vi "LastName.vi"(2 "Custom Folder":string, 3 "Extention":string="dat", 4 "User Data Folder":path) -> (0 "created path":path, 1 "String":string)   [LabVIEW 2017]
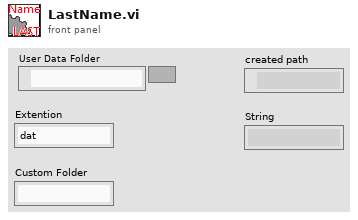
[diagram p1: front panel]
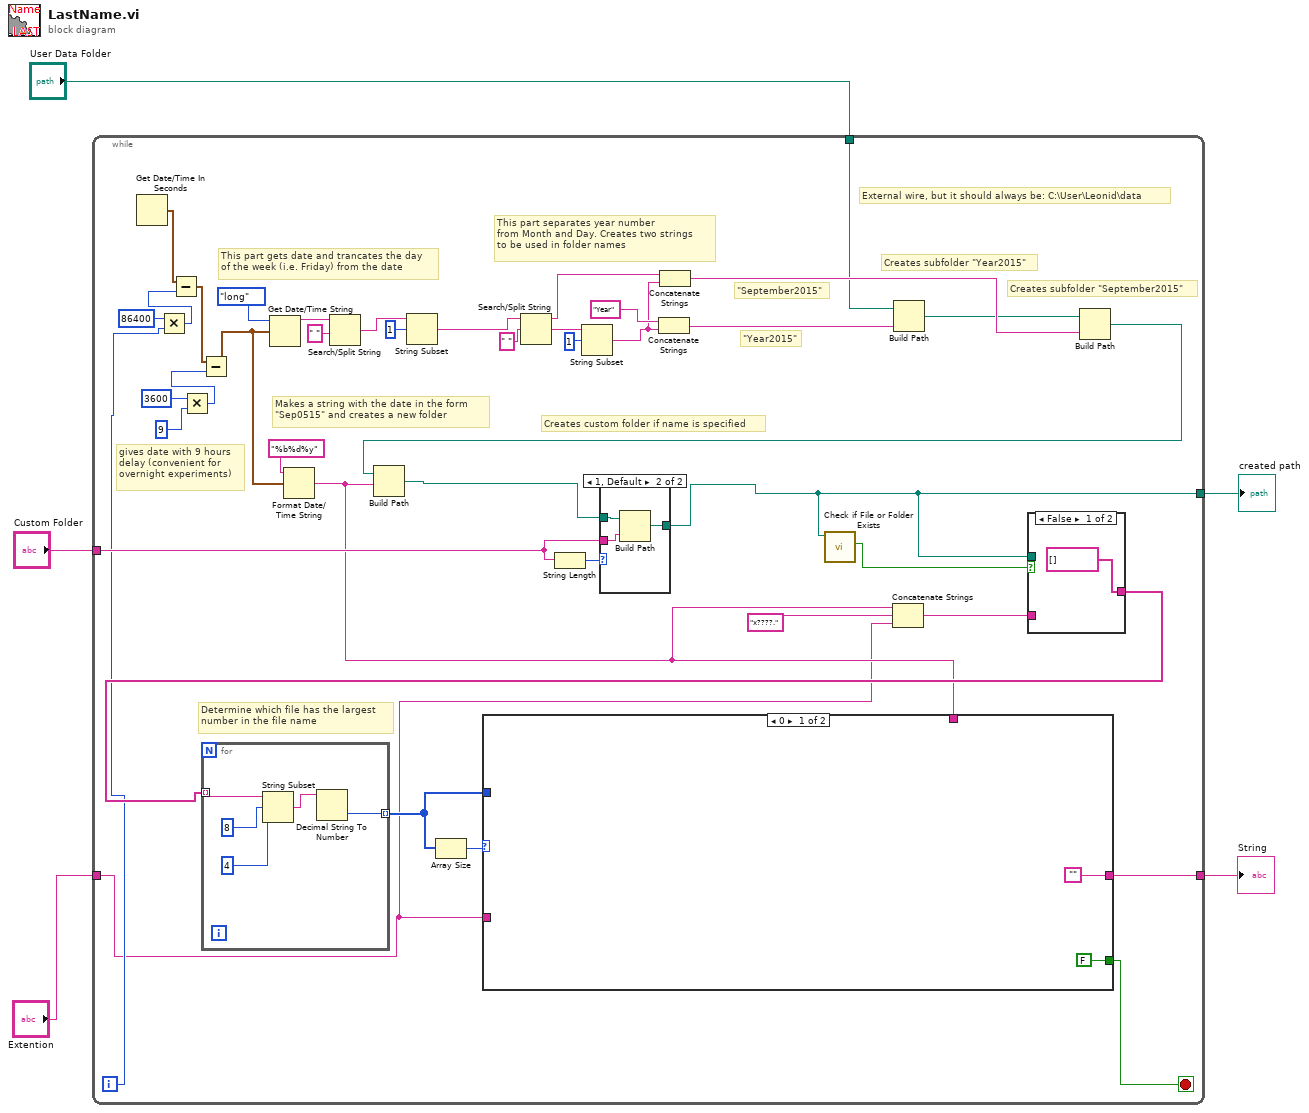
[diagram p0: block diagram]
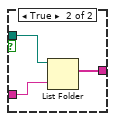
[diagram p2: hidden frame]
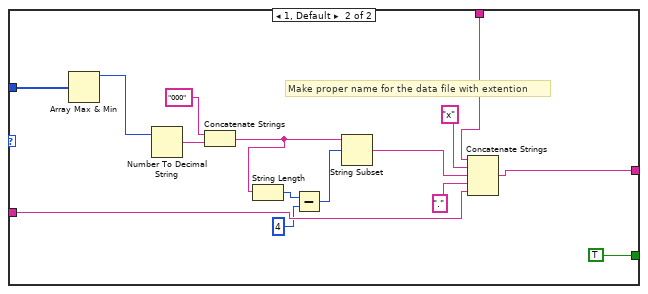
[diagram p3: hidden frame]
diagram:
  n1 = while {
    tunnel: [w6] -> w4
    tunnel: "User Data Folder" -> [w29]
    tunnel: "Custom Folder" -> [w25]
    tunnel: "Extention" -> [w11]
    tunnel: [w21] -> w1
    i -> [w16]
    stop <- w12 stop-if-true
    # "Determine which file has the largest \nnumber in the file name"
    # "External wire, but it should always be: C:\\User\\Leonid\\data"
    # "Creates custom folder if name is specified"
    # "Makes a string with the date in the form \n\"Sep0515\" and creates a new folder"
    # "Creates subfolder \"September2015\""
    # "Creates subfolder \"Year2015\""
    # "\"September2015\""
    # "\"Year2015\""
    # "This part separates year number \nfrom Month and Day. Creates two strings\nto be used in folder names"
    # "This part gets date and trancates the day \nof the week (i.e. Friday) from the date"
    # "gives date with 9 hours \ndelay (convenient for \novernight experiments)"
    n2 = Get Date/Time In Seconds() -> (seconds since 1Jan1904=w18:timestamp)
    n3 = Multiply(x=86400, y=w16) -> (x*y=w19:i32)
    n4 = Subtract(x=w18, y=w19) -> (x-y=w17:timestamp)
    n5 = Multiply(x=3600, y=9) -> (x*y=w27:i32)
    n6 = Subtract(x=w17, y=w27) -> (x-y=w24:timestamp)
    n7 = Get Date/Time String(date format (0)=enum16{"short", "long", "abbreviated"}."long", seconds (now)=w24) -> (date string=w42:string)  [unwired: 1 in, 1 out]
    n8 = Format Date/Time String(time format string (%c)="%b%d%y", seconds (now)=w24) -> (date/time string=w22:string)  [unwired: 1 in]
    n9 = Search/Split String(string=w42, search string/char (-)=" ") -> (match + rest of string=w40:string)  [unwired: 1 in, 2 out]
    n10 = String Subset(string=w40, offset (0)=1) -> (substring=w35:string)  [unwired: 1 in]
    n11 = Search/Split String(string=w35, search string/char (-)=" ") -> (substring before match=w31:string, match + rest of string=w36:string)  [unwired: 1 in, 1 out]
    n12 = String Length(string=w25) -> (length=w26:i32)
    n13 = String Subset(string=w36, offset (0)=1) -> (substring=w32:string)  [unwired: 1 in]
    n14 = Concatenate Strings("Year" ("Substring"), w32) -> (w33:string)
    n15 = Concatenate Strings(w31, w32) -> (w30:string)
    n16 = Concatenate Strings(w22, "x????.", w11) -> (w45:string)
    n17 = Build Path(base path=w29, name or relative path=w33) -> (appended path=w10:path)
    n18 = Build Path(base path=w10, name or relative path=w30) -> (appended path=w9:path)
    n19 = Build Path(base path=w9, name or relative path=w22) -> (appended path=w8:path)
    n20 = case shown="1, Default" w26 {
      tunnel: [w73 w76] -> w6
      tunnel: w8 -> [w73 w75]
      tunnel: w25 -> [_ w74]
      frame 0 {
      }
      frame 1, Default {
        n21 = Build Path(base path=w75, name or relative path=w74) -> (appended path=w76:path)
      }
    }
    n22 = call <vilib>:"Check if File or Folder Exists.vi"("path"=w6) -> ("file or folder exists?"=w7:bool)  [unwired: 8 in, 2 out]
    n23 = case shown="False" w7 {
      tunnel: w45 -> [_ w50]
      tunnel: [string[] [] w49] -> w23
      tunnel: w6 -> [_ w48]
      frame False {
      }
      frame True {
        n24 = List Folder(path=w48, pattern=w50) -> (filenames=w49:string[])  [unwired: 2 in, 3 out]
      }
    }
    n25 = for {
      tunnel: w23 -> [w72] mode=indexing
      tunnel: [w68] -> w14 mode=indexing
      n26 = String Subset(string=w72, offset (0)=8, length (rest)=4) -> (substring=w69:string)
      n27 = Decimal String To Number(string=w69) -> (number=w68:i32)  [unwired: 2 in, 1 out]
    }
    n28 = Array Size(array=w14) -> (size(s)=w13:i32)
    n29 = case shown="0" w13 {
      tunnel: w11 -> [_ w67]
      tunnel: w22 -> [_ w57]
      tunnel: ["" w56] -> w21
      tunnel: w14 -> [_ w54]
      tunnel: [FALSE TRUE] -> w12
      frame 0 {
      }
      frame 1, Default {
        # "Make proper name for the data file with extention"
        n30 = Array Max & Min(array=w54) -> (max value=w55:i32)  [unwired: 3 out]
        n31 = Number To Decimal String(number=w55) -> (decimal integer string=w66:string)  [unwired: 1 in]
        n32 = Concatenate Strings("000", w66) -> (w61:string)
        n33 = String Length(string=w61) -> (length=w64:i32)
        n34 = Subtract(x=w64, y=4) -> (x-y=w62:i32)
        n35 = String Subset(string=w61, offset (0)=w62) -> (substring=w58:string)  [unwired: 1 in]
        n36 = Concatenate Strings(w57, "x", w58, "." ("Substring"), w67) -> (w56:string)
      }
    }
  }
  "created path" <- w4
  "String" <- w1
